vi "One 32-bit Port Digital Input.vi"(2 "32-Bit DI Port":refnum<k21>="Chassis1/Mod4/DI7:0") -> (7 "Packet":u64)   [LabVIEW 2009]
uses:
  <vilib>/eio/EIONode/EIONode.xnode
  <vilib>/rvi/eio/nirviEIOImplementation/nirviEIOImplementation.xnode
  <vilib>/rvi/eio/common/nirviEmuTemplateMethod_noerrors.vi
  <vilib>/rvi/eio/common/nirviEmuClasses.ctl
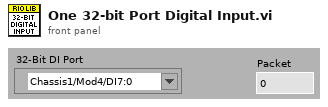
[diagram p1: front panel]
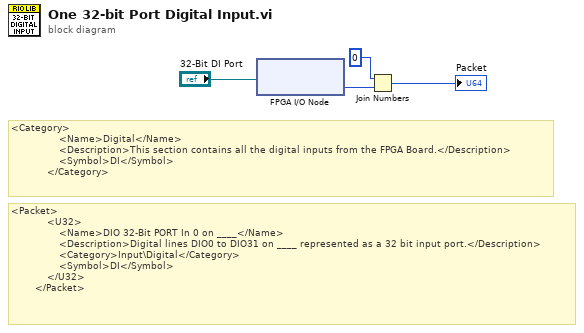
[diagram p0: block diagram]
diagram:
  # "<Packet>\n            <U32>\n                <Name>DIO 32-Bit PORT In 0 on ____</Name>\n                <Description>Digital lines DIO0 to DIO31 on ____ represented as a 32 bit input port.</Description>\n                <Category>Input\\Digital</Category>\n                <Symbol>DI</Symbol>\n            </U32>\n        </Packet>"
  # "<Category>\n                <Name>Digital</Name>\n                <Description>This section contains all the digital inputs from the FPGA Board.</Description>\n                <Symbol>DI</Symbol>\n            </Category>"
  n1 = xnode "FPGA I/O Node"("FPGA I/O In"="32-Bit DI Port") -> ("I/O Item"=w2:u32)  [unwired: 1 out]
  n2 = Join Numbers(hi=u32 0, lo=w2) -> ((hi.lo)=→"Packet":u64)
